vi "Pass.vi"(7 "Caller":string, 8 "error in (no error)":errorcluster, 10 "Assertion":string, 11 "Caraya Test Framework in":refnum<class "Caraya Test Framework.lvclass">) -> (0 "error out":errorcluster, 3 "Caraya Test Framework out":refnum<class "Caraya Test Framework.lvclass">)   [LabVIEW 2017, in "Caraya Test Framework.lvclass"]
doc: "Executes the unit test framework-specific operation to indicate a passing test."
uses:
  Caraya Test Framework.lvclass
  Caraya Adapter/Caraya Adapter.lvclass
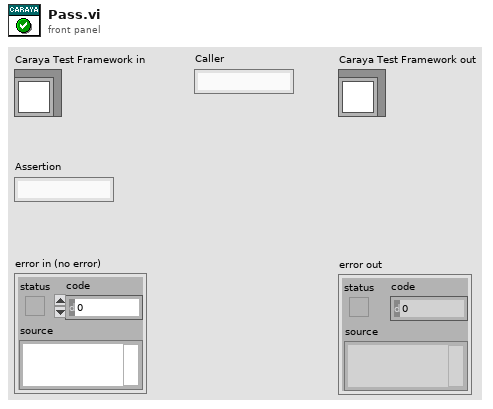
[diagram p1: front panel]
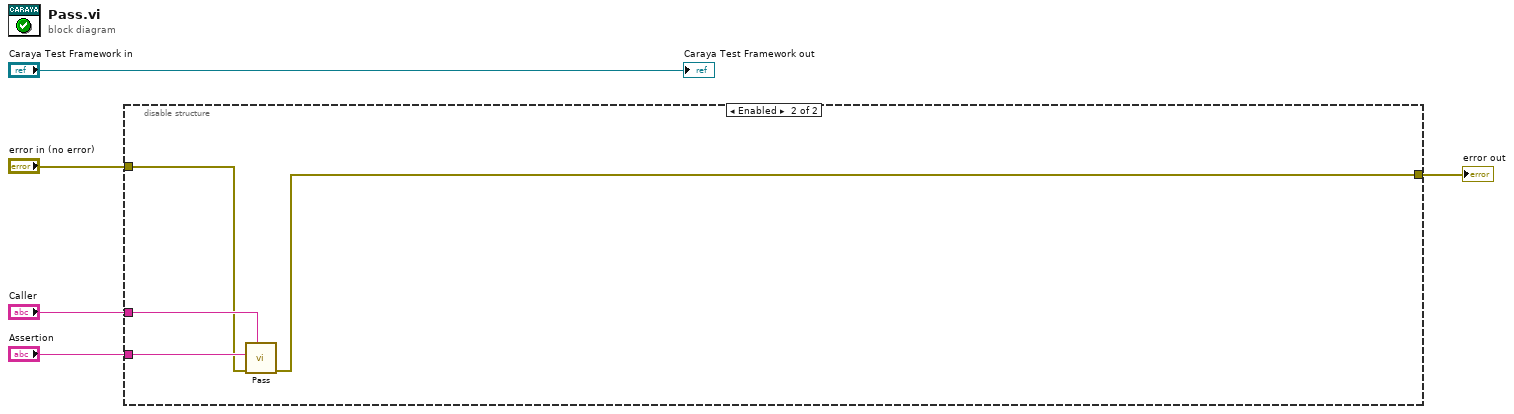
[diagram p0: block diagram]
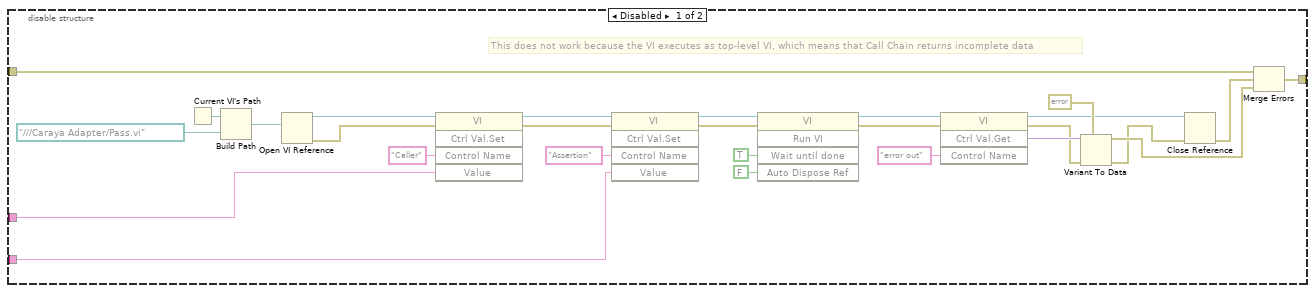
[diagram p2: hidden frame]
diagram:
  n1 = disable-structure shown="Enabled" {
    disable-tunnel: "error in (no error)" -> [w17 w34]
    disable-tunnel: [w16 w33] -> w3
    disable-tunnel: "Assertion" -> [w7 w35]
    disable-tunnel: "Caller" -> [w6 w36]
    frame Disabled {
      # "This does not work because the VI executes as top-level VI, which means that Call Chain returns incomplete data"
      n2 = Current VI's Path() -> (path=w32:path)
      n3 = Build Path(base path=w32, name or relative path=path "../../../Caraya Adapter/Pass.vi") -> (appended path=w30:path)
      n4 = Open VI Reference(vi path=w30) -> (vi reference=w29:refnum<vi>, error out=w15:errorcluster)  [unwired: 5 in]
      n5 = invoke class="VI" method="Ctrl Val.Set"(reference=w29, error in=w15, "Control Name"="Caller", "Value"=w6) -> (reference out=w27:refnum<vi>, error out=w14:errorcluster)  [unwired: 1 in, 3 out]
      n6 = invoke class="VI" method="Ctrl Val.Set"(reference=w27, error in=w14, "Control Name"="Assertion", "Value"=w7) -> (reference out=w25:refnum<vi>, error out=w13:errorcluster)  [unwired: 1 in, 3 out]
      n7 = invoke class="VI" method="Run VI"(reference=w25, error in=w13, "Wait until done"=TRUE ("Wait Until Done"), "Auto Dispose Ref"=FALSE ("Auto Dispose Reference")) -> (reference out=w22:refnum<vi>, error out=w12:errorcluster)  [unwired: 1 in, 3 out]
      n8 = invoke class="VI" method="Ctrl Val.Get"(reference=w22, error in=w12, "Control Name"="error out") -> (reference out=w18:refnum<vi>, error out=w9:errorcluster, "Get Control Value Variant"=w20:variant)  [unwired: 1 in, 1 out]
      n9 = Variant To Data(error in=w9, type=errorcluster {"status"=FALSE, "code"=0, "source"=""} ("error constant"), Variant=w20) -> (data=w10:errorcluster, error out=w8:errorcluster)
      n10 = Close Reference(reference=w18, error in (no error)=w8) -> (error out=w11:errorcluster)
      n11 = Merge Errors(w17, w11, w10) -> (w16:errorcluster)
    }
    frame Enabled {
      n12 = call "Pass.vi"("Caller"=w36, "error in (no error)"=w34, "Assertion"=w35) -> ("error out"=w33:errorcluster)  [unwired: 8 in]
    }
  }
  "error out" <- w3
  "Caraya Test Framework out" <- "Caraya Test Framework in"
